vi "Application name.vi"() -> (1 "download site":string, 2 "help site":string="http://ceeserver.cee.cornell.edu/mw24/Software/", 3 "application name":string)   [LabVIEW 2015]
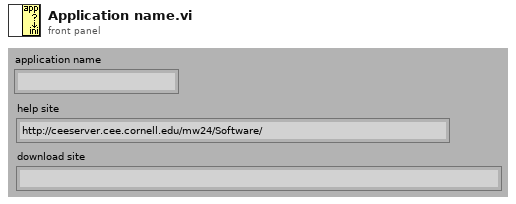
[diagram p1: front panel]
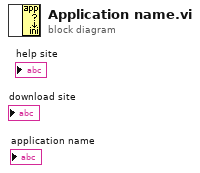
[diagram p0: block diagram]
diagram:
